vi "Get Profile Header-Footer Size.vi"() -> (0 "Footer Size":u32, 2 "Header Size":u32)   [LabVIEW 2014, in "Keyence LJ-V7000.lvlib"]
uses:
  Keyence LJ-V7000.lvlib
  Public/Clusters/Profile Header.ctl
  Public/Clusters/Profile Footer.ctl
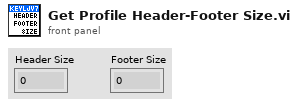
[diagram p1: front panel]
types:
  T1 = typedef "Keyence LJ-V7000.lvlib/Profile Footer.ctl" = cluster{"reserve":u32}
  T2 = typedef "Keyence LJ-V7000.lvlib/Profile Header.ctl" = cluster{"Encoder Z-in":u32, "Trigger Cnt":u32, "Encoder Cnt":u32, "reserve":u32, "reserve":u32, "reserve":u32}
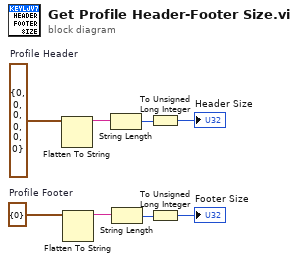
[diagram p0: block diagram]
diagram:
  w5 = T1 {"reserve"=0}  # Profile Footer
  w7 = T2 {"Encoder Z-in"=0, "Trigger Cnt"=0, "Encoder Cnt"=0, "reserve"=0, "reserve"=0, "reserve"=0}  # Profile Header
  n1 = Flatten To String(anything=w7) -> (data string=w8:string)  [unwired: 3 in, 2 out]
  n2 = Flatten To String(anything=w5) -> (data string=w6:string)  [unwired: 3 in, 2 out]
  n3 = String Length(string=w8) -> (length=w4:i32)
  n4 = String Length(string=w6) -> (length=w3:i32)
  n5 = To Unsigned Long Integer(number=w4) -> (unsigned 32bit integer=→"Header Size":u32)
  n6 = To Unsigned Long Integer(number=w3) -> (unsigned 32bit integer=→"Footer Size":u32)
